vi "Update DO (SubVI).vi"(8 "error in":errorcluster, 9 "IP Address":string[](array[string]), 10 "DO Input":T1(array[cluster])) -> (0 "error out":errorcluster)   [LabVIEW 2021]
uses:
  Controls/Host Data Cluster.ctl
  Main Engine/Controls/Main Engine CPU Info.ctl
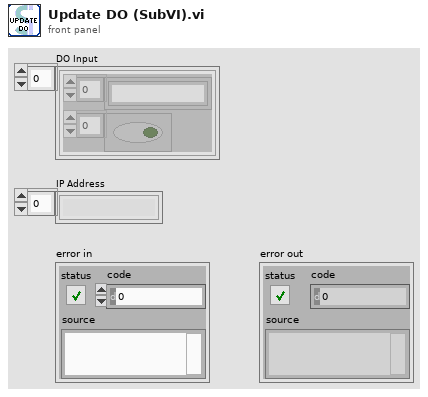
[diagram p1: front panel]
types:
  T1 = cluster{"Channel Name":string[], "Data":bool[]}[]
  T2 = typedef "Host Data Cluster.ctl" = cluster{"AI":dbl[], "DI":bool[], "DO":bool[], "Serial":string[][], "CPU":T3, "Stop":bool, "DO Channel":string[]}
  T3 = typedef "Main Engine CPU Info.ctl" = cluster{"Total Load":u32[], "Interrupt Load":u32[], "Total Physical":dbl, "Free Physical":dbl, "Primary Disk Capacity":dbl, "Primary Disk Free":dbl}
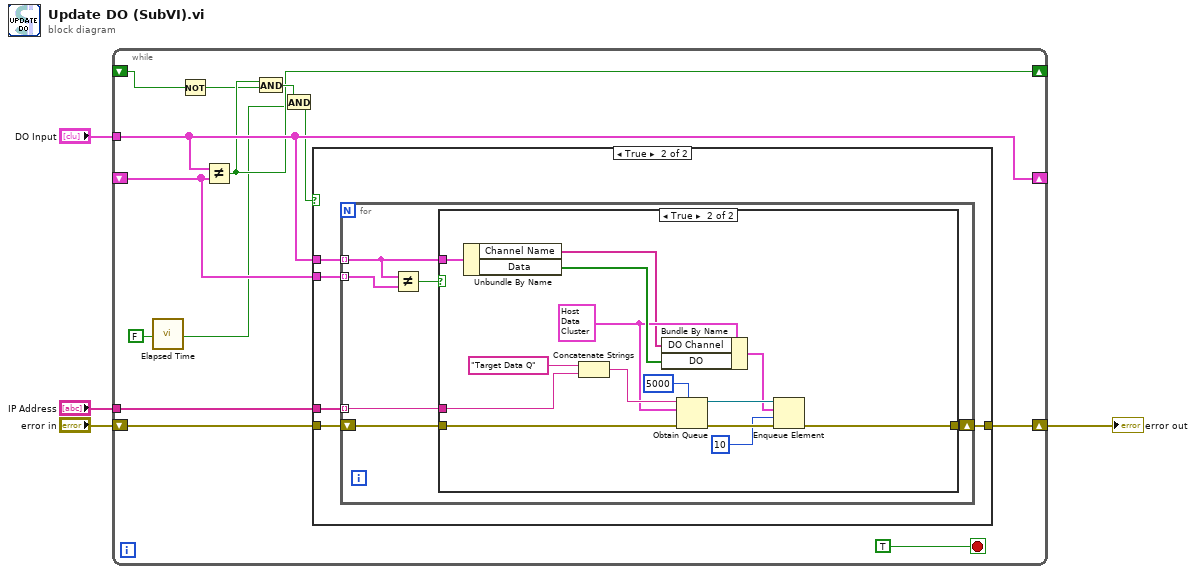
[diagram p0: block diagram]
diagram:
  n1 = while {
    shift-right: [w11] -> _
    shift-left: _ -> [w13]
    tunnel: "DO Input" -> [w11]
    shift-right: [w15] -> w4
    shift-left: "error in" -> [w16]
    tunnel: "IP Address" -> [w14]
    shift-right: [w10] -> _
    shift-left: _ -> [w8]
    stop <- TRUE stop-if-true
    n2 = call "Elapsed Time"("Auto Reset"=FALSE) -> ("Time has Elapsed"=w5:bool)  [unwired: 11 in, 7 out]
    n3 = Not(x=w8) -> (.not. x?=w9:bool)
    n4 = Not Equal?(x=w11, y=w13) -> (x != y?=w10:bool)
    n5 = And(x=w10, y=w9) -> (x .and. y?=w12:bool)
    n6 = And(x=w12, y=w5) -> (x .and. y?=w7:bool)
    n7 = case shown="True" w7 {
      tunnel: w11 -> [_ w19]
      tunnel: w13 -> [_ w23]
      tunnel: w14 -> [_ w22]
      tunnel: w16 -> [w18 w21]
      tunnel: [w18 w20] -> w15
      frame False {
      }
      frame True {
        n8 = for {
          tunnel: w19 -> [w27] mode=indexing
          tunnel: w23 -> [w29] mode=indexing
          tunnel: w22 -> [w28] mode=indexing
          shift-right: [w25] -> w20
          shift-left: w21 -> [w26]
          n9 = Not Equal?(x=w27, y=w29) -> (x != y?=w24:bool)
          n10 = case shown="True" w24 {
            tunnel: w28 -> [_ w44]
            tunnel: w27 -> [_ w43]
            tunnel: w26 -> [w30 w41]
            tunnel: [w30 w40] -> w25
            frame False {
            }
            frame True {
              w32 = T2 {"AI"=[-3.29963760152739, -3.28042607250678, -3.30275742266883, -3.28305329003257, -3.29914499819412, -3.27566424083626, -3.29520417157553, -3.26269235518028, -3.14446761533159, -3.13215254239399, -3.16088771377303, -3.13198834142664, -3.16959036650255, -3.151528257494, -3.17188918049567, -3.1431540075152, -3.2208210848143, -3.21425304324317, -3.24479443847459, -3.23132995179905, -3.24922786722435, -3.22706072451644, -3.22311989941762, -3.18896608529332, -3.07895143597999, -3.07616002028715, -3.11064221681751, -3.08551947305428, -3.12459929803547, -3.10916440827463, -3.12197208267327], "DI"=[FALSE, FALSE, FALSE, FALSE, FALSE, FALSE, FALSE, FALSE, FALSE, FALSE, FALSE, FALSE, FALSE, FALSE, FALSE, FALSE, FALSE, FALSE, FALSE, FALSE, FALSE, FALSE, FALSE, FALSE, FALSE, FALSE, FALSE, FALSE, FALSE, FALSE, FALSE, FALSE, FALSE, FALSE, FALSE, FALSE, FALSE, FALSE, FALSE, FALSE, FALSE, FALSE, FALSE, FALSE, FALSE, FALSE, FALSE, FALSE, FALSE, FALSE, FALSE, FALSE, FALSE, FALSE, FALSE, FALSE, FALSE, FALSE, FALSE, FALSE, FALSE, FALSE, FALSE, FALSE], "DO"=[], "Serial"=[], "CPU"={"Total Load"=[], "Interrupt Load"=[], "Total Physical"=0.0, "Free Physical"=0.0, "Primary Disk Capacity"=0.0, "Primary Disk Free"=0.0}, "Stop"=FALSE, "DO Channel"=[]} ("Data Out")
              n11 = Unbundle By Name(w43) -> ("Channel Name"=w31:string[], "Data"=w42:bool[])
              n12 = Concatenate Strings("Target Data Q" ("name (unnamed)"), w44) -> (w39:string)
              n13 = Bundle By Name(cluster=w32, "DO Channel"=w31, "DO"=w42) -> (w35:T2)
              n14 = Obtain Queue(max queue size (-1, unlimited)=5000, name (unnamed)=w39, element data type=w32, error in (no error)=w41) -> (queue out=w36:refnum<queue>, error out=w34:errorcluster)  [unwired: 1 in, 1 out]
              n15 = Enqueue Element(queue=w36, element=w35, timeout in ms (-1)=10, error in (no error)=w34) -> (error out=w40:errorcluster)  [unwired: 2 out]
            }
          }
        }
      }
    }
  }
  "error out" <- w4
